vi "dll.midi_get_input_device_name.vi"(8 "error in (no error)":errorcluster, 10 "Device Index":i32, 11 "LabVIEW-MIDI-XPLAT in":refnum<class "midi in.lvclass">) -> (0 "error out":errorcluster, 2 "Device Names":string, 3 "LabVIEW-MIDI-XPLAT out":refnum<class "midi in.lvclass">)   [LabVIEW 2020, in "MIDIllan.lvlib" / "midi in.lvclass"]
uses:
  midi in.lvclass
  midi in.lvclass/midi in.ctl
  MIDIllan/MIDIllan.lvlib
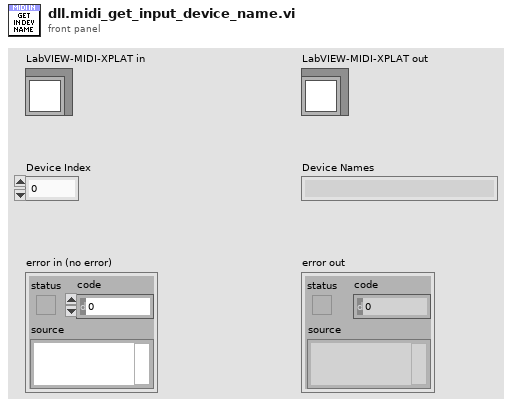
[diagram p1: front panel]
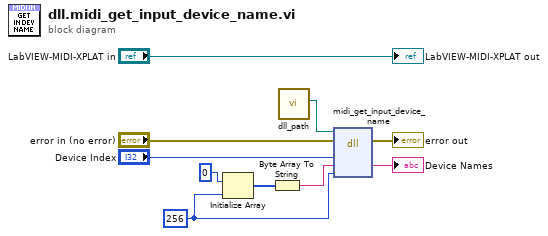
[diagram p0: block diagram]
diagram:
  w5 = 256 ("dimension size")
  n1 = Initialize Array(u8 0, w5) -> (w3:u8[])
  n2 = Byte Array To String(unsigned byte array=w3) -> (string=w6:string)
  n3 = call "dll_path.vi"() -> ("dll"=w7:path)  [unwired: 11 in]
  n4 = dll-call lib="C:/code/LabVIEW-MIDI-XPLAT/dist/TomMIDIllan_*.*" fn="midi_get_input_device_name"(path in=w7, error in="error in (no error)", "device_index"="Device Index", "buffer"=w6, "buffer_size"=w5) -> (error out=→"error out":errorcluster, "buffer"=→"Device Names":string)  [unwired: 4 in, 1 out]
  "LabVIEW-MIDI-XPLAT out" <- "LabVIEW-MIDI-XPLAT in"
